vi "Superimpose Trace Indication.vi"(6 "Line Color":u32(colorbox)=16711680, 7 "Width":dbl=0.015, 8 "error in":errorcluster, 10 "Line Data":cluster{"Line Points":T1[], "Wrap?":bool}[](array[cluster]), 11 "Image In":T2) -> (0 "error out":errorcluster, 3 "Image Out":T2)   [LabVIEW 2011]
uses:
  <vilib>/vision/Image Controls.llb/IMAQ Image.ctl
  Type Definitions/Fiducial with Source.ctl
  Vec3d Class/Vec3d Class.lvclass
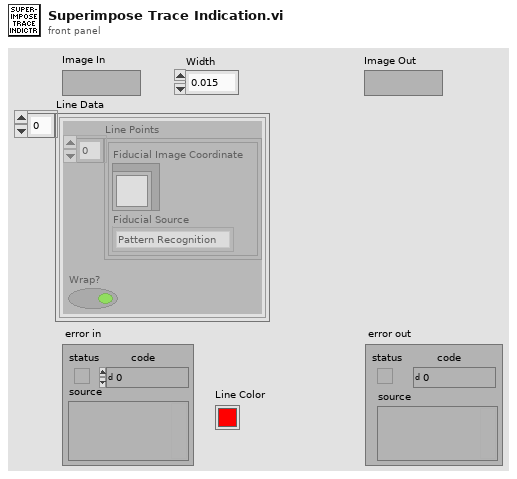
[diagram p1: front panel]
types:
  T1 = typedef "Fiducial with Source.ctl" = cluster{"Fiducial Image Coordinate":refnum<class "Vec3d Class.lvclass">, "Fiducial Source":enum16{"Pattern Recognition", "User", "Error", "Default"}}
  T2 = typedef "IMAQ Image.ctl" = refnum<image>
  T3 = enum16{"Pattern Recognition", "User", "Error", "Default"}
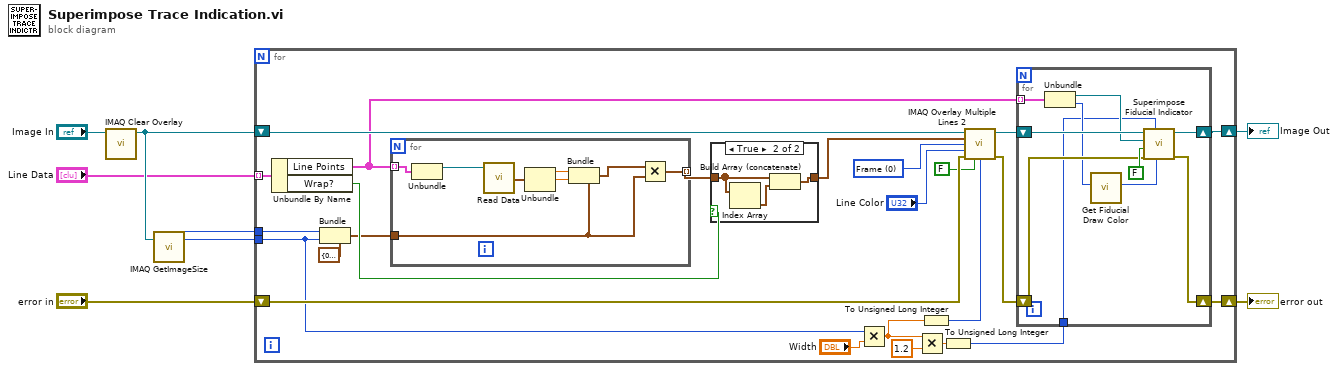
[diagram p0: block diagram]
diagram:
  n1 = call "IMAQ Clear Overlay"("Image"="Image In") -> ("Image Out"=w4:T2)  [unwired: 9 in, 1 out]
  n2 = call "IMAQ GetImageSize"("Image"=w4) -> ("Y Resolution"=w2:i32, "X Resolution"=w1:i32)  [unwired: 3 in, 1 out]
  n3 = for {
    shift-right: [w14] -> w6
    shift-left: "error in" -> [w31]
    shift-right: [w16] -> w8
    shift-left: w4 -> [w29]
    tunnel: "Line Data" -> [w27] mode=indexing
    tunnel: w2 -> [w20]
    tunnel: w1 -> [w22]
    w32 = u32 0 items=["Frame", "Fill"] ("Drawing Mode (Frame)")
    n4 = Unbundle By Name(w27) -> ("Line Points"=w13:T1[], "Wrap?"=w26:bool)
    n5 = Bundle(cluster=cluster{"X":dbl, "Y":dbl} {"X"=0.0, "Y"=0.0} ("Point Coordinates"), "X"=w22, "Y"=w20) -> (w21:cluster{"X":dbl, "Y":dbl})
    n6 = for {
      tunnel: w13 -> [w44] mode=indexing
      tunnel: w21 -> [w48]
      tunnel: [w50] -> w19 mode=indexing
      n7 = Unbundle(w44) -> ("Fiducial Image Coordinate"=w43:refnum<class "Vec3d Class.lvclass">)  [unwired: 1 out]
      n8 = call-dynamic "Read Data.vi"("Vec3d Class in"=w43) -> ("Data"=w49:cluster{"X":dbl, "Y":dbl, "Z":dbl})  [unwired: 8 in, 2 out]
      n9 = Unbundle(w49) -> ("X"=w47:dbl, "Y"=w46:dbl)  [unwired: 1 out]
      n10 = Bundle(cluster=w48, "X"=w47, "Y"=w46) -> (w45:cluster{"X":dbl, "Y":dbl})
      n11 = Multiply(x=w45, y=w48) -> (x*y=w50:cluster{"X":dbl, "Y":dbl})
    }
    n12 = case shown="True" w26 {
      tunnel: w19 -> [w51 w54]
      tunnel: [w51 w52] -> w18
      frame False {
      }
      frame True {
        n13 = Index Array(array=w54) -> (element=w53:cluster{"X":dbl, "Y":dbl})  [unwired: 1 in]
        n14 = Build Array (concatenate)(w54, w53) -> (w52:cluster{"X":dbl, "Y":dbl}[])
      }
    }
    n15 = Multiply(x=w20, y="Width") -> (x*y=w12:dbl)
    n16 = Multiply(x=w12, y=1.2) -> (x*y=w10:dbl)
    n17 = To Unsigned Long Integer(number=w12) -> (unsigned 32bit integer=w24:u32)
    n18 = To Unsigned Long Integer(number=w10) -> (unsigned 32bit integer=w9:u32)
    n19 = call "IMAQ Overlay Multiple Lines 2"("Image"=w29, "Line End Points"=w18, "Drawing Mode (Frame)"=w32, "Color"="Line Color", "error in (no error)"=w31, "Maintain Width?"=FALSE, "Width"=w24) -> ("Image Out"=w17:T2, "error out"=w15:errorcluster)  [unwired: 7 in]
    n20 = for {
      tunnel: w13 -> [w37] mode=indexing
      shift-right: [w40] -> w16
      shift-left: w17 -> [w41]
      shift-right: [w38] -> w14
      shift-left: w15 -> [w39]
      tunnel: w9 -> [w33]
      n21 = Unbundle(w37) -> ("Fiducial Image Coordinate"=w36:refnum<class "Vec3d Class.lvclass">, "Fiducial Source"=w35:T3)
      n22 = call "Get Fiducial Draw Color.vi"("Fiducial Source"=w35) -> ("Grid Line Color"=w34:u32)  [unwired: 10 in]
      n23 = call "Superimpose Fiducial Indicator.vi"("Marker Color"=w34, "size(pixels)"=w33, "error in"=w39, "Clear Previous Overlay"=FALSE, "Fiducial Image Coordinates"=w36, "Image In"=w41) -> ("error out"=w38:errorcluster, "Image Out"=w40:T2)  [unwired: 4 in]
    }
  }
  "Image Out" <- w8
  "error out" <- w6
